vi "Tolerance to color converter.vi"(4 "Tolerance":T1) -> (1 "Tolerance to  color":u32(colorbox))   [LabVIEW 2018]
uses:
  Ramon Taboada/ProyectoPrueba/Tolerance--control.ctl
  Resistor Band Colors/Resistor Band Colors.lvlib
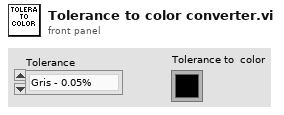
[diagram p1: front panel]
types:
  T1 = typedef "Tolerance--control.ctl" = enum16{"Gris - 0.05%", "Violeta - 0.1%", "Azul - 0.25%", "Verde - 0.5%", "Marron - 1%", "Rojo - 2%", "Oro - 5%", "Plata - 10%", "Ninguno - 20%"}
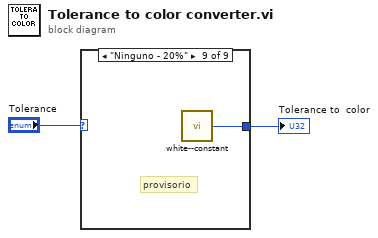
[diagram p0: block diagram]
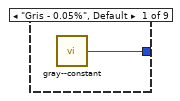
[diagram p2: hidden frame]
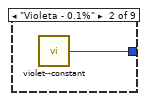
[diagram p3: hidden frame]
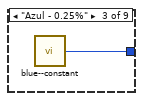
[diagram p4: hidden frame]
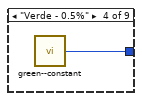
[diagram p5: hidden frame]
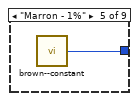
[diagram p6: hidden frame]
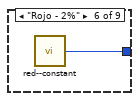
[diagram p7: hidden frame]
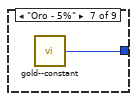
[diagram p8: hidden frame]
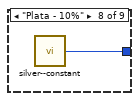
[diagram p9: hidden frame]
diagram:
  n1 = case shown="\"Ninguno - 20%\"" "Tolerance" {
    tunnel: [w3 w4 w5 w6 w7 w8 w9 w10 w11] -> w1
    frame "Gris - 0.05%", Default {
      n2 = call "gray--constant.vi"() -> ("gray"=w3:u32)  [unwired: 5 in]
    }
    frame "Violeta - 0.1%" {
      n3 = call "violet--constant.vi"() -> ("violet"=w4:u32)  [unwired: 5 in]
    }
    frame "Azul - 0.25%" {
      n4 = call "blue--constant.vi"() -> ("blue"=w5:u32)  [unwired: 5 in]
    }
    frame "Verde - 0.5%" {
      n5 = call "green--constant.vi"() -> ("green"=w6:u32)  [unwired: 5 in]
    }
    frame "Marron - 1%" {
      n6 = call "brown--constant.vi"() -> ("brown"=w7:u32)  [unwired: 5 in]
    }
    frame "Rojo - 2%" {
      n7 = call "red--constant.vi"() -> ("red"=w8:u32)  [unwired: 5 in]
    }
    frame "Oro - 5%" {
      n8 = call "gold--constant.vi"() -> ("Gold"=w9:u32)  [unwired: 5 in]
    }
    frame "Plata - 10%" {
      n9 = call "silver--constant.vi"() -> ("silver"=w10:u32)  [unwired: 5 in]
    }
    frame "Ninguno - 20%" {
      # "provisorio"
      n10 = call "white--constant.vi"() -> ("white"=w11:u32)  [unwired: 5 in]
    }
  }
  "Tolerance to  color" <- w1
